vi "Untokenize.vi"(9 "tokens":string[](array[string]), 10 "line terminator (\\n)":string="\n", 11 "delimiter (=)":string="=") -> (3 "string out":string)   [LabVIEW 2010]
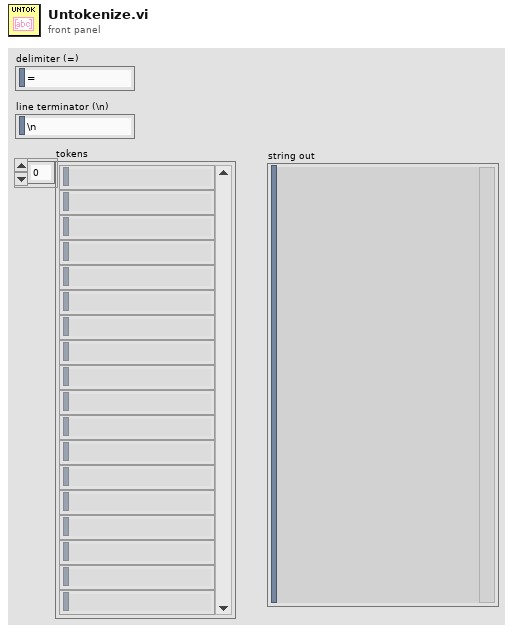
[diagram p1: front panel]
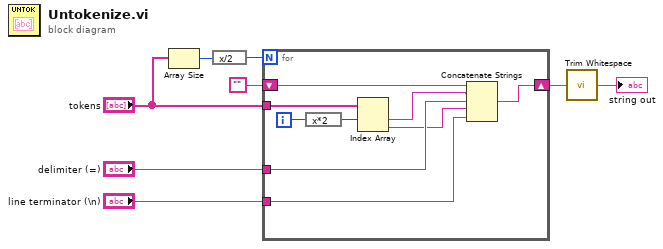
[diagram p0: block diagram]
diagram:
  n1 = Array Size(array="tokens") -> (size(s)=w4:i32)
  n2 = expression code="x/2"(w4) -> (w3:i32)
  n3 = for {
    N: w3 -> [_]
    shift-right: [w9] -> w2
    shift-left: "" -> [w17]
    tunnel: "tokens" -> [w16]
    tunnel: "delimiter (=)" -> [w12]
    tunnel: "line terminator (\\n)" -> [w10]
    i -> [w15]
    n4 = expression code="x*2"(w15) -> (w14:i32)
    n5 = Index Array(array=w16, index #1=w14) -> (element #1=w13:string, element #2=w11:string)  [unwired: 1 in]
    n6 = Concatenate Strings(w17, w13, w12, w11, w10) -> (w9:string)
  }
  n7 = call <vilib>:"Trim Whitespace.vi"("string"=w2) -> ("trimmed string"=→"string out":string)  [unwired: 1 in]
